vi "Set Channel.vi"(8 "error in (no error)":errorcluster, 10 "channelParameter":T1={"channel"=1, "gain"=enum."10", "input"=enum."DIFF", "shunt"=enum."Open", "couple"=enum."DC", "filter"=enum."ON"} {"channel" min=1 max=8 step=1}, 11 "VISA Refnum in":refnum<visa-resource-name>="COM1") -> (0 "error out":errorcluster, 3 "VISA Refnum out":refnum<visa-resource-name>)   [LabVIEW 2019, in "KH7008.lvlib"]
uses:
  KH7008.lvlib
  typedefs/channelProperties--Cluster.ctl
  typedefs/channel--numeric.ctl
  typedefs/gain--enum.ctl
  typedefs/Input--Enum.ctl
  typedefs/shunt--enum.ctl
  typedefs/couple--Enum.ctl
  typedefs/Filter--Enum.ctl
panel:
  out "Response":string
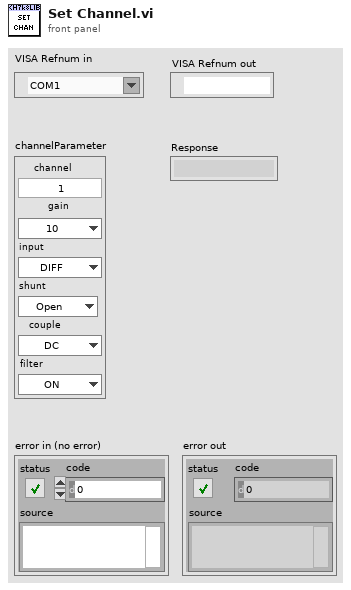
[diagram p1: front panel]
types:
  T1 = typedef "KH7008.lvlib/channelProperties--Cluster.ctl" = cluster{"channel":T2, "gain":T3, "input":T4, "shunt":T5, "couple":T6, "filter":T7}
  T2 = typedef "KH7008.lvlib/channel--numeric.ctl" = u16
  T3 = typedef "KH7008.lvlib/gain--enum.ctl" = enum16{"1", "10", "100", "1000"}
  T4 = typedef "KH7008.lvlib/input--enum.ctl" = enum16{"OFF", "SE+", "SE-", "DIFF"}
  T5 = typedef "KH7008.lvlib/shunt--enum.ctl" = enum16{"Open", "50", "500", "5k", "50k", "10M"}
  T6 = typedef "KH7008.lvlib/couple--enum.ctl" = enum16{"AC", "DC"}
  T7 = typedef "KH7008.lvlib/filter--enum.ctl" = enum16{"OFF", "ON"}
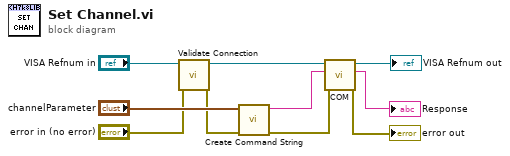
[diagram p0: block diagram]
diagram:
  n1 = call "Validate Connection.vi"("error in (no error)"="error in (no error)", "VISA Refnum in"="VISA Refnum in") -> ("error out"=w1:errorcluster, "VISA Refnum out"=w2:refnum<visa-resource-name>)  [unwired: 8 in]
  n2 = call "Create Command String.vi"("error in (no error)"=w1, "Channel Params"="channelParameter") -> ("error out"=w8:errorcluster, "Command string"=w5:string)  [unwired: 8 in]
  n3 = call "COM.vi"("error in (no error)"=w8, "Command"=w5, "VISA Refnum in"=w2) -> ("error out"=→"error out":errorcluster, "Response"=→"Response":string, "VISA Refnum out"=→"VISA Refnum out":refnum<visa-resource-name>)  [unwired: 6 in]
